vi "Controller Send State.vi"(8 "error in (no error)":errorcluster, 11 "RDS Controller Actor in":refnum<class "RDS Controller Actor.lvclass">) -> (0 "error out":errorcluster, 3 "RDS Controller Actor out":refnum<class "RDS Controller Actor.lvclass">)   [LabVIEW 2015, in "RDS Controller Actor.lvlib" / "RDS Controller Actor.lvclass"]
uses:
  RDS Controller Actor.lvclass
  Libraries/RDS Child Messages/Controller State Message/Controller State.lvclass
  Libraries/RDS Framework/RDS Message ID.ctl
  RDS Controller Actor.lvclass/RDS Controller Actor.ctl
  Libraries/RDS Framework/RDS Message Class/RDS Message.lvclass/RDS Message.ctl
  Libraries/RDS Child Messages/Controller State Message/Controller State.lvclass/Controller State.ctl
  Libraries/RDS Framework/RDS Message Class/RDS Message.lvclass
  Libraries/RDS Child Messages/RDS Child Messages.lvlib
  RDS Parent Actor/RDS Parent Actor/RDS Parent Actor.lvclass
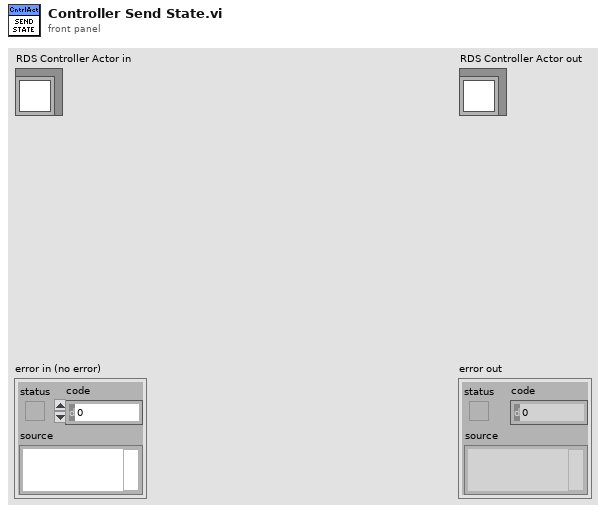
[diagram p1: front panel]
types:
  T1 = typedef "RDS Child Messages.lvlib/RDS Message ID.ctl" = enum16{"RDS Hello World", "String Message", "AIP_Status", "AIP_Command", "GPS_Data", "MCB_Command", "MCB_Status", "Compass_Data", "Depth_Data", "Battery_Data", "Contoller_State", "Set_Mag_Dev", "BTB_Shutdown", "State_Sample_Request", "State_Sample", "PID_Gains_Set", "Helm_Limiter_Set", "Helm_Heading_Command", "Helm_Steering_Command", "Helm_Status", "Controller_Message", "AIP_Set_Min_Depth", "Mission_Controller_State", "Mission_Upload", "Mission_Set_Op_and_Run", "Mission_Settings_Set"}
  T2 = typedef "RDS Controller Actor.lvlib/Controller.ctl" = enum16{"Idle", "Local Remote Control", "Shore Remote Control", "Mission Control"}
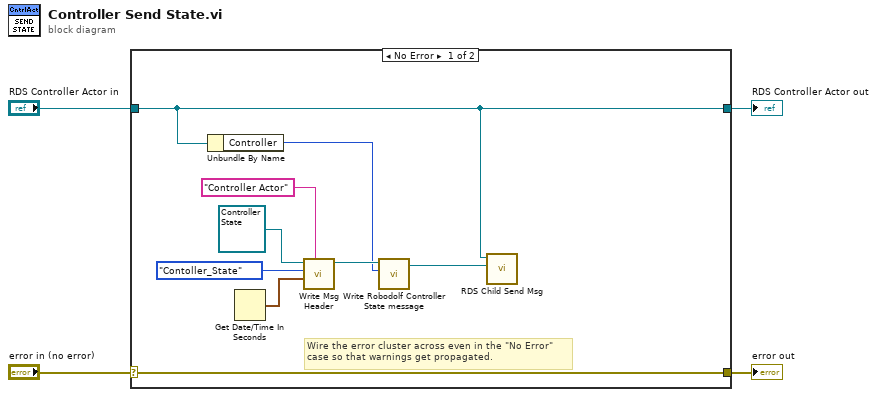
[diagram p0: block diagram]
diagram:
  n1 = case shown="No Error" "error in (no error)" {
    selector: "error in (no error)" -> [w13 w15]
    tunnel: [w13 w15] -> w3
    tunnel: [w7 w14] -> w1
    tunnel: "RDS Controller Actor in" -> [w7 w14]
    frame No Error {
      # "Wire the error cluster across even in the \"No Error\"\ncase so that warnings get propagated."
      n2 = Unbundle By Name(w7) -> ("Controller"=w5:T2)
      n3 = Get Date/Time In Seconds() -> (seconds since 1Jan1904=w11:timestamp)
      n4 = call "Write Msg Header.vi"("Sender Name"="Controller Actor", "Time Stamp"=w11, "Msg ID"=RDS_Message_ID."Contoller_State", "RDS Message in"=refnum<class "Controller State.lvclass"> refnum ("RDS Child Messages.lvlib:Controller State.lvclass")) -> ("RDS Message out"=w8:refnum<class "Controller State.lvclass">)  [unwired: 6 in, 1 out]
      n5 = call "Write Robodolf Controller State message.vi"("Controller"=w5, "Controller State in"=w8) -> ("Controller State out"=w6:refnum<class "Controller State.lvclass">)  [unwired: 8 in, 1 out]
      n6 = call "RDS Child Send Msg.vi"("RDS Message"=w6, "RDS Parent Actor in"=w7) -> ()  [unwired: 8 in, 2 out]
    }
    frame Error {
    }
  }
  "error out" <- w3
  "RDS Controller Actor out" <- w1
